vi "Keithley 2450 Output List and Acquire.vi"() -> ()   [LabVIEW 2025]
doc: "Outputs a sequence of voltages based on a list and takes readings at each point."
uses:
  Public/Data/Read (Multiple Points).vi
  Keithley 2450.lvlib
panel:
  out "Waveform Graph":dbl[][](graph)
  in  "Source Mode  (0: Voltage)":u16(ring) items=["Voltage", "Current"]
  in  "Output List":dbl[](array[numeric])=[0.1, 0.2, 0.3]
  in  "VISA resource name":refnum<visa-resource-name>
  in  "Limit  Level (0.1)":dbl=0.1
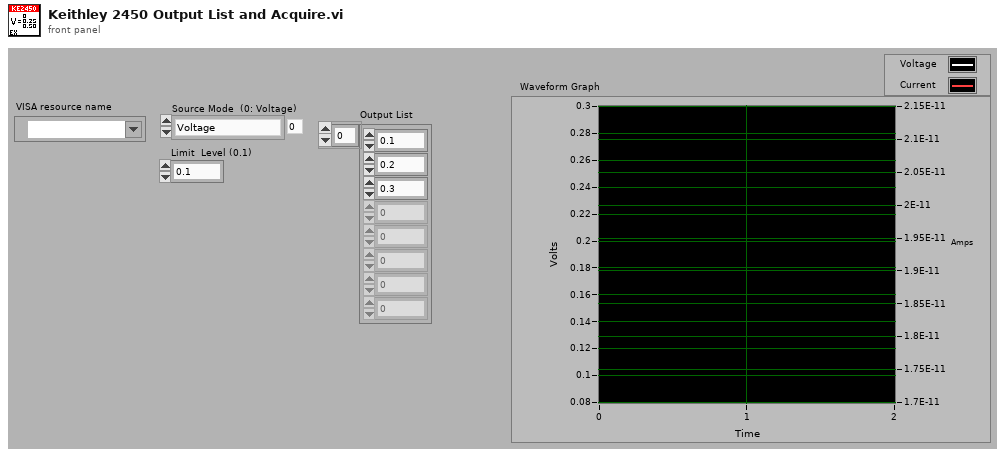
[diagram p1: front panel]
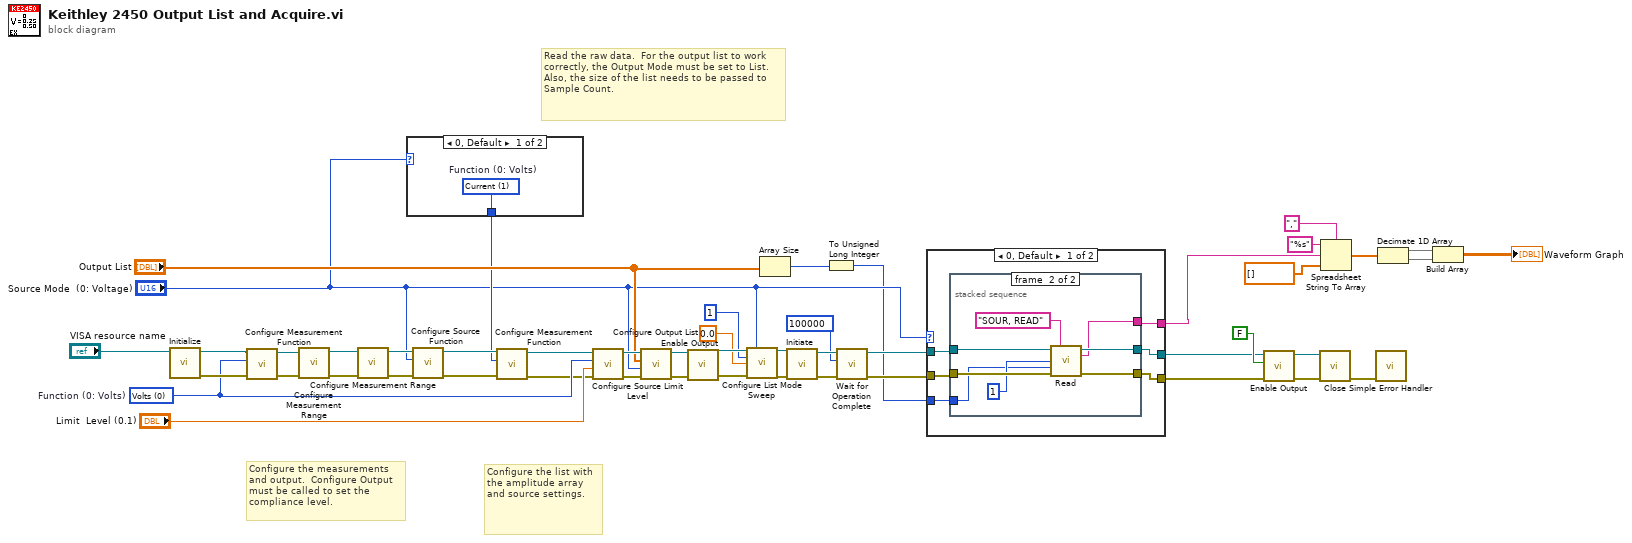
[diagram p0: block diagram]
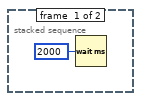
[diagram p2: hidden frame]
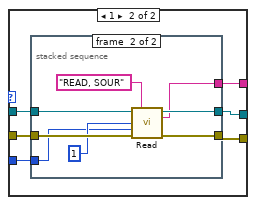
[diagram p3: hidden frame]
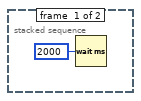
[diagram p4: hidden frame]
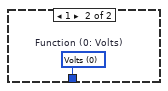
[diagram p5: hidden frame]
diagram:
  w35 = u16 0 items=["Volts", "Current", "Resistance"]  # Function (0: Volts)
  # "Read the raw data.  For the output list to work correctly, the Output Mode must be set to List.  Also, the size of the list needs to be passed to Sample Count."
  # "Configure the list with the amplitude array and source settings."
  # "Configure the measurements and output.  Configure Output must be called to set the compliance level."
  n1 = call "Initialize.vi"("VISA resource name"="VISA resource name") -> ("error out"=w41:errorcluster, "VISA resource name out"=w39:refnum<visa-resource-name>)  [unwired: 9 in]
  n2 = call "Configure Measurement Function.vi"("error in (no error)"=w41, "Function (0: Volts)"=w35, "VISA resource name"=w39) -> ("error out"=w40:errorcluster, "VISA resource name out"=w38:refnum<visa-resource-name>)  [unwired: 7 in]
  n3 = call "Configure Measurement Range.vi"("error in (no error)"=w40, "VISA resource name"=w38) -> ("error out"=w49:errorcluster, "VISA resource name out"=w48:refnum<visa-resource-name>)  [unwired: 8 in]
  n4 = call "Configure Measurement Range.vi"("error in (no error)"=w49, "VISA resource name"=w48) -> ("error out"=w37:errorcluster, "VISA resource name out"=w36:refnum<visa-resource-name>)  [unwired: 8 in]
  n5 = case shown="0, Default" "Source Mode  (0: Voltage)" {
    tunnel: [w50 w51] -> w8
    frame 0, Default {
      w50 = u16 1 items=["Volts", "Current", "Resistance"]  # Function (0: Volts)
    }
    frame 1 {
      w51 = u16 0 items=["Volts", "Current", "Resistance"]  # Function (0: Volts)
    }
  }
  n6 = call "Configure Source Function.vi"("error in (no error)"=w37, "Function (0: Volts)"="Source Mode  (0: Voltage)", "VISA resource name"=w36) -> ("error out"=w9:errorcluster, "VISA resource name out"=w12:refnum<visa-resource-name>)  [unwired: 7 in]
  n7 = call "Configure Measurement Function.vi"("error in (no error)"=w9, "Function (0: Volts)"=w8, "VISA resource name"=w12) -> ("error out"=w10:errorcluster, "VISA resource name out"=w11:refnum<visa-resource-name>)  [unwired: 7 in]
  n8 = call "Configure Source Limit Level.vi"("error in (no error)"=w10, "Source Limit (1.0)"="Limit  Level (0.1)", "Function (0: Volts)"=w35, "VISA resource name"=w11) -> ("error out"=w33:errorcluster, "VISA resource name out"=w34:refnum<visa-resource-name>)  [unwired: 6 in]
  n9 = call "Configure Output List.vi"("error in (no error)"=w33, "Source Mode  (0: Voltage)"="Source Mode  (0: Voltage)", "Output List"="Output List", "VISA resource name"=w34) -> ("error out"=w44:errorcluster, "VISA resource name out"=w45:refnum<visa-resource-name>)  [unwired: 6 in]
  n10 = call "Enable Output.vi"("error in (no error)"=w44, "VISA resource name"=w45) -> ("error out"=w32:errorcluster, "VISA resource name out"=w31:refnum<visa-resource-name>)  [unwired: 8 in]
  n11 = call "Configure List Mode Sweep.vi"("VISA resource name"=w31, "Source Mode  (0: Voltage)"="Source Mode  (0: Voltage)", "Start Index"=u32 1, "Delay (0)"=0.0 ("Delay (-1)"), "error in (no error)"=w32) -> ("VISA resource name out"=w28:refnum<visa-resource-name>, "error out"=w27:errorcluster)  [unwired: 9 in]
  n12 = Array Size(array="Output List") -> (size(s)=w25:i32)
  n13 = call "Initiate.vi"("error in (no error)"=w27, "VISA resource name"=w28) -> ("error out"=w14:errorcluster, "VISA resource name out"=w15:refnum<visa-resource-name>)  [unwired: 8 in]
  n14 = To Unsigned Long Integer(number=w25) -> (unsigned 32bit integer=w1:u32)
  n15 = call "Wait for Operation Complete.vi"("error in (no error)"=w14, "Timeout (10000 ms)"=100000, "VISA resource name"=w15) -> ("error out"=w6:errorcluster, "VISA resource name out"=w7:refnum<visa-resource-name>)  [unwired: 7 in]
  n16 = case shown="0, Default" "Source Mode  (0: Voltage)" {
    tunnel: w7 -> [w57 w72]
    tunnel: w6 -> [w56 w71]
    tunnel: [w55 w69] -> w5
    tunnel: [w54 w68] -> w4
    tunnel: w1 -> [w53 w70]
    tunnel: [w52 w67] -> w3
    frame 0, Default {
      n17 = stacked-sequence {
        tunnel: [_ w66] -> w55
        tunnel: [_ w65] -> w54
        tunnel: w57 -> [_ w63]
        tunnel: w56 -> [_ w62]
        tunnel: [_ w61] -> w52
        tunnel: w53 -> [_ w59]
        frame #0 {
          n18 = Wait (ms)(milliseconds to wait=u32 2000) -> ()  [unwired: 1 out]
        }
        frame #1 {
          n19 = call-poly "Read.vi"("VISA resource name"=w63, "Buffer Elements"="SOUR, READ", "Start Index (1)"=1, "End Index (1)"=w59, "error in (no error)"=w62) -> ("VISA resource name out"=w66:refnum<visa-resource-name>, "Data out"=w61:string, "error out"=w65:errorcluster)  [unwired: 8 in]
        }
      }
    }
    frame 1 {
      n20 = stacked-sequence {
        tunnel: [_ w81] -> w69
        tunnel: [_ w80] -> w68
        tunnel: w72 -> [_ w78]
        tunnel: w71 -> [_ w77]
        tunnel: [_ w76] -> w67
        tunnel: w70 -> [_ w74]
        frame #0 {
          n21 = Wait (ms)(milliseconds to wait=u32 2000) -> ()  [unwired: 1 out]
        }
        frame #1 {
          n22 = call-poly "Read.vi"("VISA resource name"=w78, "Buffer Elements"="READ, SOUR", "Start Index (1)"=1, "End Index (1)"=w74, "error in (no error)"=w77) -> ("VISA resource name out"=w81:refnum<visa-resource-name>, "Data out"=w76:string, "error out"=w80:errorcluster)  [unwired: 8 in]
        }
      }
    }
  }
  n23 = call "Enable Output.vi"("error in (no error)"=w4, "Enable Output (T: Enable)"=FALSE, "VISA resource name"=w5) -> ("error out"=w43:errorcluster, "VISA resource name out"=w42:refnum<visa-resource-name>)  [unwired: 7 in]
  n24 = call "Close.vi"("error in (no error)"=w43, "VISA resource name"=w42) -> ("error out"=w46:errorcluster)  [unwired: 9 in]
  n25 = Spreadsheet String To Array(delimiter (Tab)=",", format string="%s", spreadsheet string=w3, array type (2D Dbl)=dbl[] []) -> (array=w21:dbl[])
  n26 = call <vilib>:"Simple Error Handler.vi"("error in (no error)"=w46) -> ()  [unwired: 4 in, 5 out]
  n27 = Decimate 1D Array(w21) -> (w20:dbl[], w19:dbl[])
  n28 = Build Array(w20, w19) -> (→"Waveform Graph":dbl[][])
